vi "nCrproj.vi"() -> ()   [LabVIEW 2024]
panel:
  out "nPr":dbl
  out "nCr":dbl
  in  "r":dbl
  in  "n":dbl
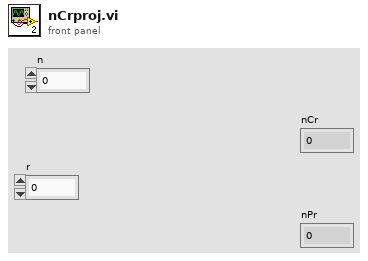
[diagram p1: front panel]
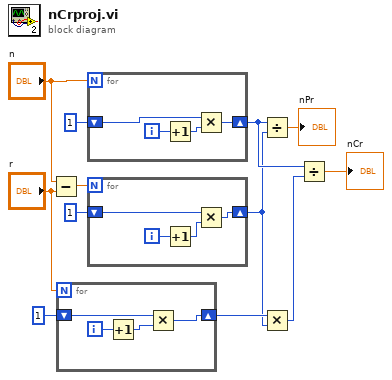
[diagram p0: block diagram]
diagram:
  n1 = Subtract(x="n", y="r") -> (x-y=w7:dbl)
  n2 = for {
    N: "r" -> [_]
    shift-right: [w16] -> w5
    shift-left: 1 -> [w15]
    i -> [w14]
    n3 = Increment(x=w14) -> (x+1=w13:i32)
    n4 = Multiply(x=w15, y=w13) -> (x*y=w16:i32)
  }
  n5 = for {
    N: "n" -> [_]
    shift-right: [w20] -> w2
    shift-left: 1 -> [w19]
    i -> [w18]
    n6 = Increment(x=w18) -> (x+1=w17:i32)
    n7 = Multiply(x=w19, y=w17) -> (x*y=w20:i32)
  }
  n8 = for {
    N: w7 -> [_]
    shift-right: [w24] -> w1
    shift-left: 1 -> [w23]
    i -> [w22]
    n9 = Increment(x=w22) -> (x+1=w21:i32)
    n10 = Multiply(x=w23, y=w21) -> (x*y=w24:i32)
  }
  n11 = Divide(x=w2, y=w1) -> (x/y=→"nPr":dbl)
  n12 = Multiply(x=w5, y=w1) -> (x*y=w4:i32)
  n13 = Divide(x=w2, y=w4) -> (x/y=→"nCr":dbl)
